vi "digital clock.vi"() -> ()   [LabVIEW 2012]
uses:
  black bg digit.ctl
  vertical.ctl
  horizontal.ctl
panel:
  out "Seconds":T1[](array[typedef])
  out "Minutes":T1[](array[typedef])
  out "Hours":T1[](array[typedef])
  in  "Stop Button":bool
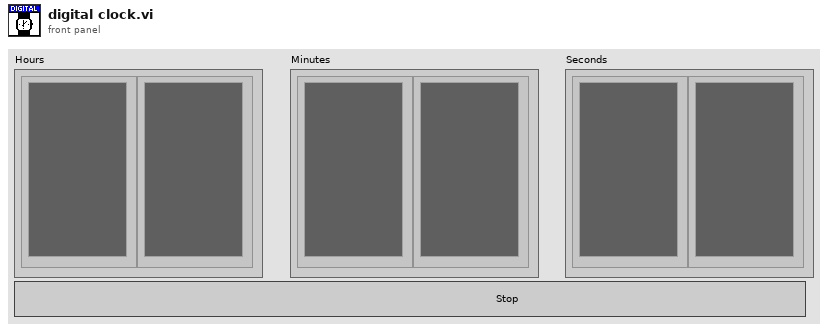
[diagram p1: front panel]
types:
  T1 = typedef "black bg digit.ctl" = cluster{"V1":T2, "V2":T2, "H1":T3, "H2":T3, "V3":T2, "V4":T2, "H3":T3}
  T2 = typedef "vertical.ctl" = bool
  T3 = typedef "horizontal.ctl" = bool
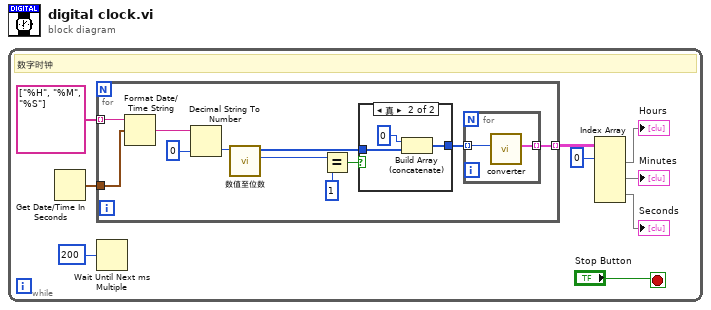
[diagram p0: block diagram]
diagram:
  n1 = while {
    stop <- "Stop Button" stop-if-true
    # "数字时钟"
    n2 = Get Date/Time In Seconds() -> (seconds since 1Jan1904=w8:timestamp)
    n3 = for {
      tunnel: w8 -> [w20]
      tunnel: [w13] -> w5 mode=indexing
      tunnel: string[] ["%H", "%M", "%S"] -> [w12] mode=indexing
      n4 = Format Date/Time String(time format string (%c)=w12, seconds (now)=w20) -> (date/time string=w19:string)  [unwired: 1 in]
      n5 = Decimal String To Number(string=w19, default (0L)=u8 0 ("默认(0 I32)")) -> (number=w11:u8)  [unwired: 1 in, 1 out]
      n6 = call-poly "数值至位数.vi"("输入数值"=w11) -> ("总位数"=w18:i32, "位数数组"=w15:u8[])  [unwired: 8 in, 1 out]
      n7 = Equal?(x=w18, y=1) -> (x = y?=w16:bool)
      n8 = case shown="真" w16 {
        tunnel: w15 -> [w23 w25]
        tunnel: [w23 w24] -> w14
        frame False {
        }
        frame True {
          n9 = Build Array (concatenate)(u8 0 ("元素"), w25) -> (w24:u8[])
        }
      }
      n10 = for {
        tunnel: w14 -> [w22] mode=indexing
        tunnel: [w21] -> w13 mode=indexing
        n11 = call "converter.vi"("Digit"=w22) -> ("Digit"=w21:T1)  [unwired: 7 in, 1 out]
      }
    }
    n12 = Wait Until Next ms Multiple(millisecond multiple=u32 200) -> ()  [unwired: 1 out]
    n13 = Index Array(array=w5, index (row) #1=0 ("索引 (行)")) -> (element #1=→"Hours":T1[], element #2=→"Minutes":T1[], element #3=→"Seconds":T1[])  [unwired: 5 in]
  }
